vi "Create Table.vi"(7 "Location":T1={"Sheet Name"="", "Name"="", "Display Name"="", "Range or Cell Address"="A1:B2"}, 8 "error in":errorcluster, 9 "Values":variant[][](array[variant]), 10 "Header Names":string[](array[string]), 11 "SpreadsheetDoc in":refnum<k24>) -> (0 "error out":errorcluster, 2 "Table":refnum<k24>, 3 "SpreadsheetDoc out":refnum<k24>)   [LabVIEW 2019, in "Open Xml.lvlib"]
uses:
  Open Xml.lvlib
  D:/git/Open-Xml-LabVIEW/Source/DocumentFormat.OpenXml.dll
  DocumentFormat.OpenXml.dll
  D:/git/Open-Xml-LabVIEW/Source/DocumentFormat.OpenXml.Framework.dll
  DocumentFormat.OpenXml.Framework.dll
  D:/git/Open-Xml-LabVIEW/Source/OpenXmlGenericsWrapper.dll
  OpenXmlGenericsWrapper.dll
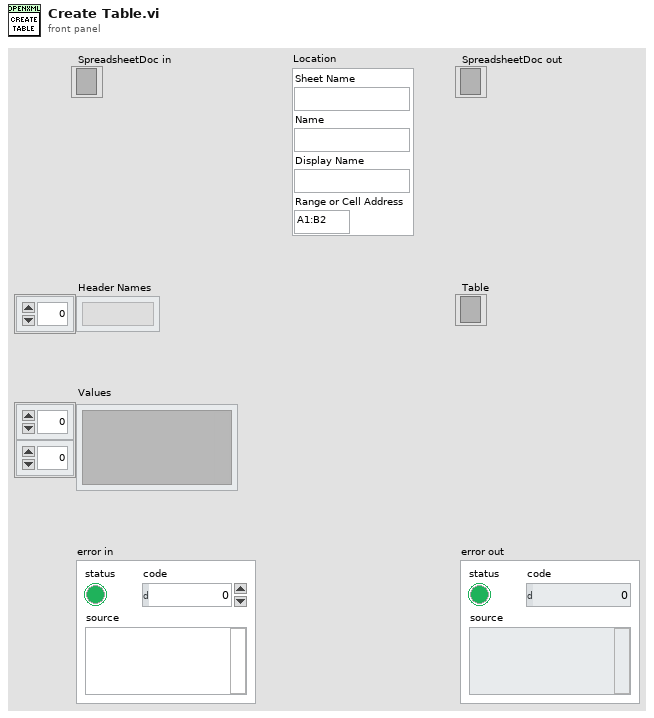
[diagram p1: front panel]
types:
  T1 = cluster{"Sheet Name":string, "Name":string, "Display Name":string, "Range or Cell Address":string}
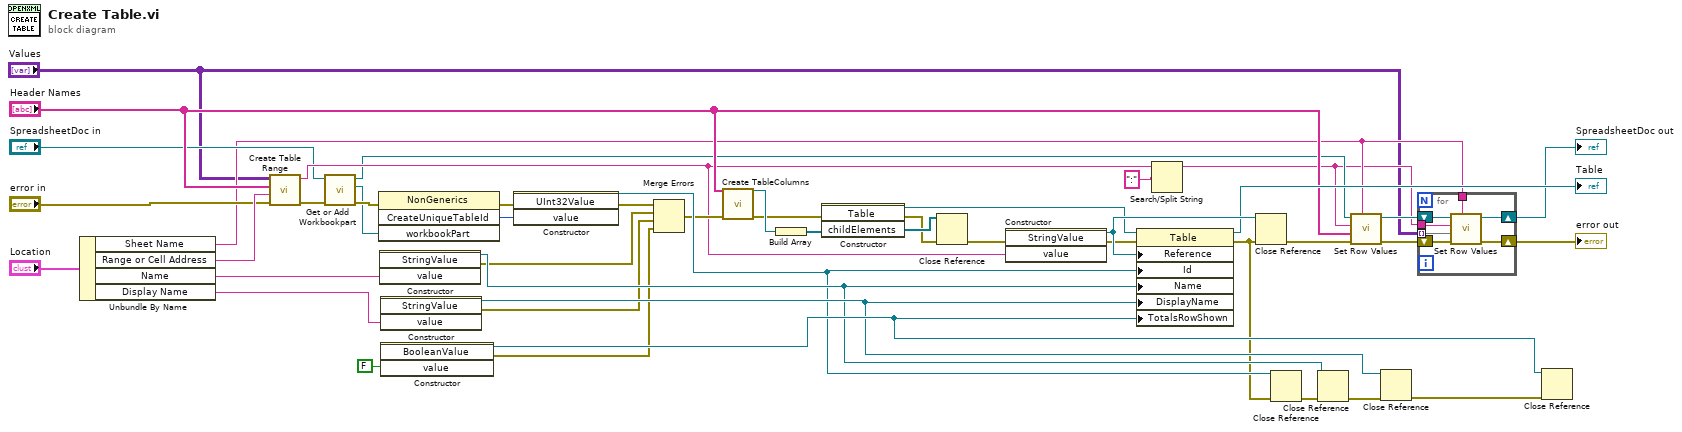
[diagram p0: block diagram]
diagram:
  n1 = Unbundle By Name("Location") -> ("Sheet Name"=w3:string, "Range or Cell Address"=w17:string, "Name"=w20:string, "Display Name"=w19:string)
  n2 = call "Create Table Range.vi"("error in"="error in", "Range or Cell Address"=w17, "Header Names"="Header Names", "Values"="Values") -> ("error out"=w16:errorcluster, "Table Range"=w13:string)  [unwired: 6 in]
  n3 = call "Get or Add Workbookpart.vi"("error in"=w16, "SpreadsheetDoc in"="SpreadsheetDoc in") -> ("error out"=w11:errorcluster, "WorkbookPart"=w8:refnum<k24>, "SpreadsheetDoc out"=w9:refnum<k24>)  [unwired: 7 in]
  n4 = invoke class="NonGenerics" method="CreateUniqueTableId"(error in=w11, "workbookPart"=w8) -> (error out=w32:errorcluster, "CreateUniqueTableId"=w33:u32)  [unwired: 2 in, 2 out]
  n5 = constructor class="StringValue"("value"=w20) -> (reference out=w44:refnum<k24>, error out=w36:errorcluster)  [unwired: 3 in, 2 out]
  n6 = constructor class="StringValue"("value"=w19) -> (reference out=w45:refnum<k24>, error out=w35:errorcluster)  [unwired: 3 in, 2 out]
  n7 = constructor class="BooleanValue"("value"=FALSE) -> (reference out=w46:refnum<k24>, error out=w40:errorcluster)  [unwired: 3 in, 2 out]
  n8 = constructor class="UInt32Value"(error in=w32, "value"=w33) -> (reference out=w43:refnum<k24>, error out=w28:errorcluster)  [unwired: 2 in, 2 out]
  n9 = Merge Errors(w28, w36, w35, w40) -> (w27:errorcluster)
  n10 = call "Create TableColumns.vi"("error in"=w27, "Header Names"="Header Names") -> ("error out"=w25:errorcluster, "TableColumns"=w26:refnum<k24>)  [unwired: 8 in]
  n11 = Build Array(w26) -> (w31:refnum<k24>[])
  n12 = constructor class="Table"(error in=w25, "childElements"=w31) -> (reference out=w30:refnum<k24>, error out=w23:errorcluster, "childElements"=w47:refnum<k24>[])  [unwired: 2 in, 1 out]
  n13 = Close Reference(reference=w47, error in (no error)=w23) -> (error out=w22:errorcluster)
  n14 = constructor class="StringValue"(error in=w22, "value"=w13) -> (reference out=w42:refnum<k24>, error out=w24:errorcluster)  [unwired: 2 in, 2 out]
  n15 = property class="Table"(reference=w30, error in=w24, "Reference"=w42, "Id"=w43, "Name"=w44, "DisplayName"=w45, "TotalsRowShown"=w46) -> (reference out=→"Table":refnum<k24>, error out=w41:errorcluster)
  n16 = Search/Split String(string=w13, search string/char (-)=":") -> (substring before match=w2:string)  [unwired: 1 in, 2 out]
  n17 = Close Reference(reference=w42, error in (no error)=w41) -> (error out=w14:errorcluster)
  n18 = Close Reference(reference=w43, error in (no error)=w41) -> (error out=w34:errorcluster)
  n19 = Close Reference(reference=w44, error in (no error)=w34) -> (error out=w37:errorcluster)
  n20 = call "Set Row Values.vi"("Sheet Name"=w3, "error in"=w14, "Values"="Header Names", "Cell Address"=w2, "SpreadsheetDoc"=w9) -> ("error out"=w7:errorcluster, "SpreadsheetDoc out"=w5:refnum<k24>)  [unwired: 5 in]
  n21 = Close Reference(reference=w45, error in (no error)=w37) -> (error out=w38:errorcluster)
  n22 = for {
    shift-right: [w53] -> w6
    shift-left: w7 -> [w54]
    shift-right: [w51] -> w4
    shift-left: w5 -> [w52]
    tunnel: w3 -> [w50]
    tunnel: w2 -> [w49]
    tunnel: "Values" -> [w48] mode=indexing
    n23 = call "Set Row Values.vi"("Sheet Name"=w50, "error in"=w54, "Values"=w48, "Cell Address"=w49, "SpreadsheetDoc"=w52) -> ("error out"=w53:errorcluster, "SpreadsheetDoc out"=w51:refnum<k24>)  [unwired: 5 in]
  }
  "error out" <- w6
  "SpreadsheetDoc out" <- w4
  n24 = Close Reference(reference=w46, error in (no error)=w38) -> ()  [unwired: 1 out]
